vi "Binary U8 to Digital.vi"(7 "Compress Data (T: Enable)":bool=TRUE, 8 "error in (no error)":errorcluster, 11 "Binary Array":i32[](array[numeric])) -> (0 "error out":errorcluster, 3 "Digital Data":digitaldata)   [LabVIEW 2017, in "Tektronix DPO MSO 2000 4000 Series.lvlib"]
doc: "Converts a binary array of unsigned integers to a digital waveform or set of digital data."
uses:
  Tektronix DPO MSO 2000 4000 Series.lvlib
  <vilib>/Waveform/DTblOps.llb/DTbl Compress Digital.vi
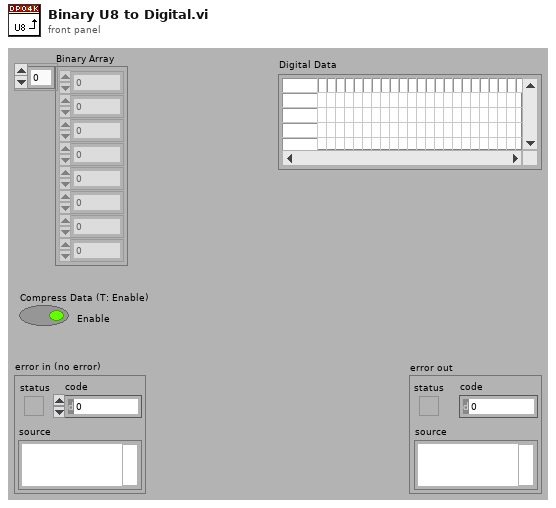
[diagram p1: front panel]
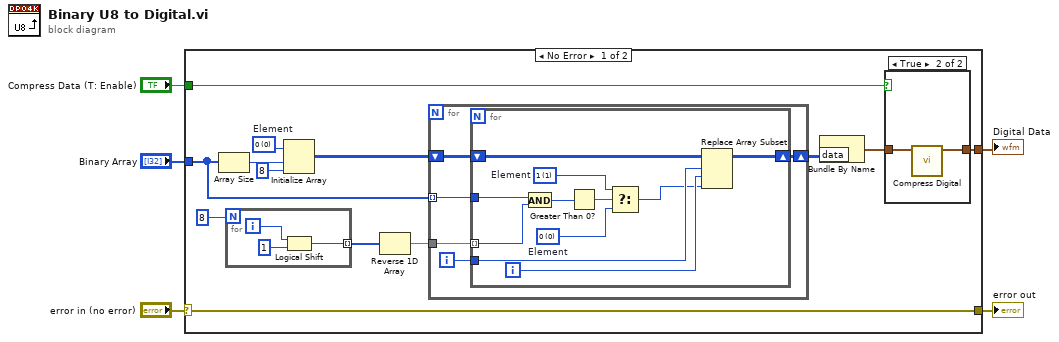
[diagram p0: block diagram]
diagram:
  n1 = case shown="No Error" "error in (no error)" {
    selector: "error in (no error)" -> [w6 w41]
    tunnel: "Compress Data (T: Enable)" -> [w7 _]
    tunnel: "Binary Array" -> [w12 _]
    tunnel: [w8 _] -> w3
    tunnel: [w6 w41] -> w1
    frame No Error {
      w16 = u16 0 items=["0", "1", "Z", "L", "H", "X", "T", "V"]  # Element
      n2 = Array Size(array=w12) -> (size(s)=w18:i32)
      n3 = for {
        N: 8 ("dimension size") -> [_]
        tunnel: [w38] -> w14 mode=indexing
        i -> [w40]
        n4 = Logical Shift(y=w40, x=1) -> (x << y=w38:i32)
      }
      n5 = Initialize Array(w16, w18, 8 ("dimension size")) -> (w13:u16[][])
      n6 = Reverse 1D Array(array=w14) -> (reversed array=w11:i32[])
      n7 = for {
        shift-right: [w25] -> w10
        shift-left: w13 -> [w26]
        tunnel: w12 -> [w24] mode=indexing
        tunnel: w11 -> [w23]
        i -> [w22]
        n8 = for {
          shift-right: [w36] -> w25
          shift-left: w26 -> [w37]
          tunnel: w24 -> [w33]
          tunnel: w23 -> [w32] mode=indexing
          tunnel: w22 -> [w34]
          i -> [w35]
          w27 = u16 0 items=["0", "1", "Z", "L", "H", "X", "T", "V"]  # Element
          w28 = u16 1 items=["0", "1", "Z", "L", "H", "X", "T", "V"]  # Element
          n9 = And(x=w33, y=w32) -> (x .and. y?=w31:i32)
          n10 = Greater Than 0?(x=w31) -> (x > 0?=w29:bool)
          n11 = Select(t=w28, s=w29, f=w27) -> (s? t:f=w30:u16)
          n12 = Replace Array Subset(array=w37, new element=w30, index (row)=w34, index (col)=w35) -> (w36:u16[][])
        }
      }
      n13 = Bundle By Name("data"=w10) -> (w9:digitaldata)  [unwired: 1 in]
      n14 = case shown="True" w7 {
        tunnel: w9 -> [w19 w21]
        tunnel: [w19 w20] -> w8
        frame False {
        }
        frame True {
          n15 = call-poly <vilib>:"Compress Digital.vi"("uncompressed digital data"=w21) -> ("compressed digital data"=w20:digitaldata)  [unwired: 9 in, 1 out]
        }
      }
    }
    frame Error {
    }
  }
  "Digital Data" <- w3
  "error out" <- w1
